vi "Notebook Saved Global.vi"() -> ()   [LabVIEW 2019, in "Notebook.lvlib"]
uses:
  Notebook.lvlib
panel:
  out "Beep on Error?":bool=TRUE
  in  "Saved Notebook Path":path
  out "First opening?":bool=TRUE
  out "Saved Notebook?":bool
  # "TRUE until the Notebook is first opened. This is used to clear the backup file at the beginning of a session"
  # "Whenever the Notebook content is modified, this flag is set to FALSE.\nUsed to format the dialog window following the \"close window\" action."
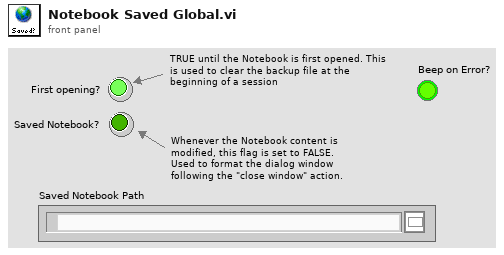
[diagram p1: front panel]
diagram:
